vi "Configure Sweep Characteristics.vi"(0 "VISA resource name":refnum<visa-resource-name>, 1 "Sweep Direction (0: Up)":u16(ring) items=["Up", "Down"], 2 "Sweep Type (0: Step)":u16(ring) items=["Step", "List", "Ramp"], 5 "Sweep Mode (0: Off)":u16(ring) items=["Off", "Frequency", "Power", "Frequency and Power"], 7 "Enable Manual Mode (F:Disable)":bool, 9 "Manual Point (1)":i32=1, 11 "error in (no error)":errorcluster, 12 "Manual Frequency (100 kHz)":dbl=100000.0, 13 "Enable Retrace (T:Enable)":bool=TRUE) -> (4 "VISA resource name out":refnum<visa-resource-name>, 15 "error out":errorcluster)   [LabVIEW 2018, in "Agilent PSG MXG Series.lvlib"]
doc: "Configures the sweep type, sweep direction, sweep mode and retrace state of the sweep functions."
uses:
  Agilent PSG MXG Series.lvlib
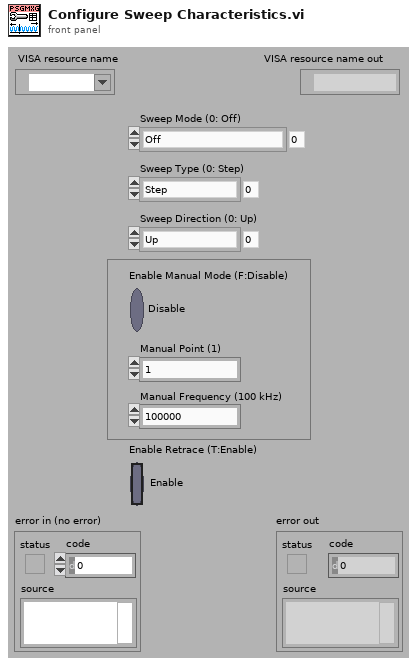
[diagram p1: front panel]
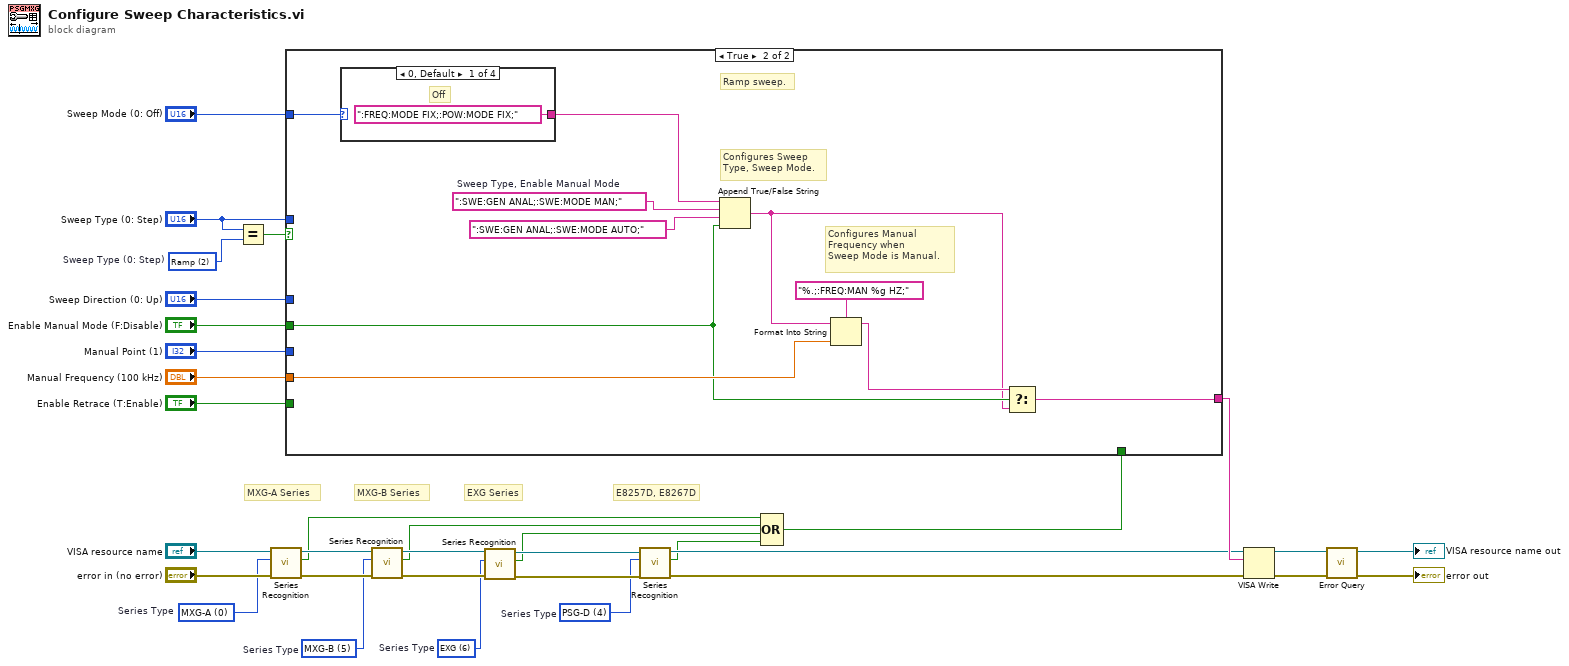
[diagram p0: block diagram]
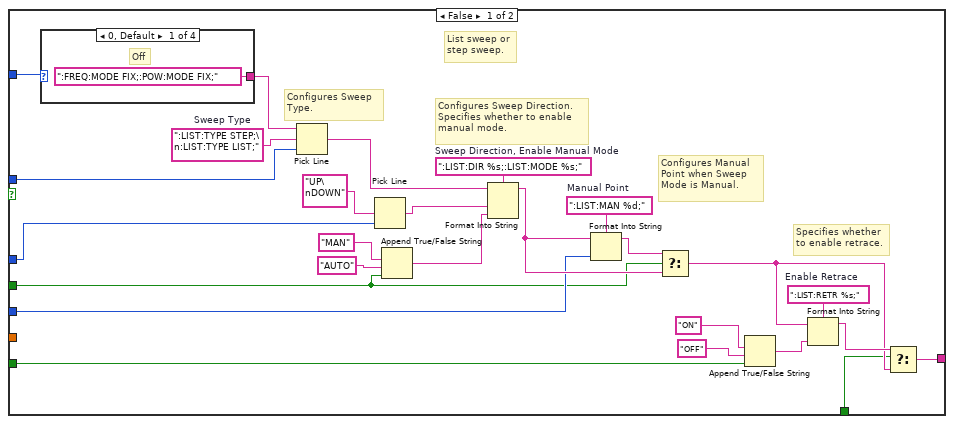
[diagram p2: hidden frame]
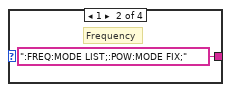
[diagram p3: hidden frame]
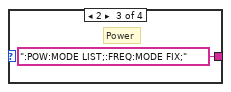
[diagram p4: hidden frame]
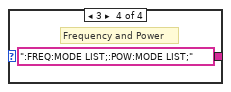
[diagram p5: hidden frame]
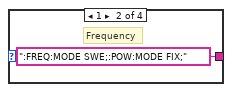
[diagram p6: hidden frame]
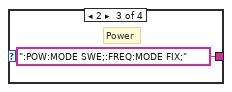
[diagram p7: hidden frame]
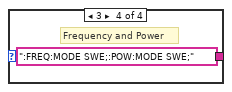
[diagram p8: hidden frame]
diagram:
  w6 = u16 6 items=["MXG-A", "PSG", "PSG-A", "PSG-C", "PSG-D", "MXG-B", "EXG"]  # Series Type
  w7 = u16 5 items=["MXG-A", "PSG", "PSG-A", "PSG-C", "PSG-D", "MXG-B", "EXG"]  # Series Type
  w8 = u16 4 items=["MXG-A", "PSG", "PSG-A", "PSG-C", "PSG-D", "MXG-B", "EXG"]  # Series Type
  w15 = u16 0 items=["MXG-A", "PSG", "PSG-A", "PSG-C", "PSG-D", "MXG-B", "EXG"]  # Series Type
  w33 = 2 items=["Step", "List", "Ramp"]  # Sweep Type (0: Step)
  # "EXG Series"
  # "MXG-B Series"
  # "E8257D, E8267D"
  # "MXG-A Series"
  n1 = Equal?(x="Sweep Type (0: Step)", y=w33) -> (x = y?=w32:bool)
  n2 = call "Series Recognition.vi"("error in (no error)"="error in (no error)", "Series Type (0: MXG)"=w15, "VISA resource name"="VISA resource name") -> ("error out"=w13:errorcluster, "Is Series Correct"=w2:bool, "VISA resource name out"=w14:refnum<visa-resource-name>)  [unwired: 1 in, 5 out]
  n3 = call "Series Recognition.vi"("error in (no error)"=w13, "Series Type (0: MXG)"=w7, "VISA resource name"=w14) -> ("error out"=w10:errorcluster, "Is Series Correct"=w3:bool, "VISA resource name out"=w12:refnum<visa-resource-name>)  [unwired: 1 in, 5 out]
  n4 = call "Series Recognition.vi"("error in (no error)"=w10, "Series Type (0: MXG)"=w6, "VISA resource name"=w12) -> ("error out"=w9:errorcluster, "Is Series Correct"=w4:bool, "VISA resource name out"=w11:refnum<visa-resource-name>)  [unwired: 1 in, 5 out]
  n5 = call "Series Recognition.vi"("error in (no error)"=w9, "Series Type (0: MXG)"=w8, "VISA resource name"=w11) -> ("error out"=w21:errorcluster, "Is Series Correct"=w5:bool, "VISA resource name out"=w22:refnum<visa-resource-name>)  [unwired: 1 in, 5 out]
  n6 = Compound Arithmetic op=OR(w2, w3, w4, w5) -> (w1:bool)
  n7 = case shown="True" w32 {
    tunnel: "Sweep Type (0: Step)" -> [w58 _]
    tunnel: "Sweep Direction (0: Up)" -> [w54 _]
    tunnel: "Enable Manual Mode (F:Disable)" -> [w36 w65]
    tunnel: "Manual Point (1)" -> [w42 _]
    tunnel: "Manual Frequency (100 kHz)" -> [_ w72]
    tunnel: [w46 w70] -> w26
    tunnel: "Enable Retrace (T:Enable)" -> [w50 _]
    tunnel: "Sweep Mode (0: Off)" -> [w40 w69]
    tunnel: w1 -> [w34 _]
    frame False {
      w45 = ":LIST:MAN %d;"  # Manual Point
      w52 = ":LIST:RETR %s;"  # Enable Retrace
      w56 = ":LIST:DIR %s;:LIST:MODE %s;"  # Sweep Direction, Enable Manual Mode
      w59 = ":LIST:TYPE STEP;\n:LIST:TYPE LIST;"  # Sweep Type
      # "Specifies whether\nto enable retrace."
      # "Configures Manual\nPoint when Sweep\nMode is Manual."
      # "Configures Sweep Direction.\nSpecifies whether to enable\nmanual mode."
      # "Configures Sweep\nType."
      # "List sweep or\nstep sweep."
      n8 = case shown="0, Default" w40 {
        tunnel: [":FREQ:MODE FIX;:POW:MODE FIX;" ":FREQ:MODE LIST;:POW:MODE FIX;" ":POW:MODE LIST;:FREQ:MODE FIX;" ":FREQ:MODE LIST;:POW:MODE LIST;"] -> w39
        frame 0, Default {
          # "Off"
        }
        frame 1 {
          # "Frequency"
        }
        frame 2 {
          # "Power"
        }
        frame 3 {
          # "Frequency and Power"
        }
      }
      n9 = Pick Line(string ("")=w39, multi-line string=w59, line index=w58) -> (output string=w57:string)
      n10 = Pick Line(multi-line string="UP\nDOWN", line index=w54) -> (output string=w53:string)  [unwired: 1 out]
      n11 = Append True/False String(1:w36, 2:"AUTO" ("false string"), 3:"MAN" ("true string")) -> (0:w35:string)  [unwired: 1 out]
      n12 = Format Into String(format string=w56, initial string=w57, w53, w35) -> (resulting string=w43:string)  [unwired: 1 in, 1 out]
      n13 = Format Into String(format string=w45, initial string=w43, w42) -> (resulting string=w44:string)  [unwired: 1 in, 1 out]
      n14 = Select(t=w44, s=w36, f=w43) -> (s? t:f=w41:string)
      n15 = Append True/False String(1:w50, 2:"OFF" ("false string"), 3:"ON" ("true string")) -> (0:w51:string)  [unwired: 1 out]
      n16 = Format Into String(format string=w52, initial string=w41, w51) -> (resulting string=w47:string)  [unwired: 1 in, 1 out]
      n17 = Select(t=w47, s=w34, f=w41) -> (s? t:f=w46:string)
    }
    frame True {
      w68 = ":SWE:GEN ANAL;:SWE:MODE MAN;"  # Sweep Type, Enable Manual Mode
      # "Configures Manual\nFrequency when\nSweep Mode is Manual."
      # "Configures Sweep\nType, Sweep Mode."
      # "Ramp sweep."
      n18 = case shown="0, Default" w69 {
        tunnel: [":FREQ:MODE FIX;:POW:MODE FIX;" ":FREQ:MODE SWE;:POW:MODE FIX;" ":POW:MODE SWE;:FREQ:MODE FIX;" ":FREQ:MODE SWE;:POW:MODE SWE;"] -> w66
        frame 0, Default {
          # "Off"
        }
        frame 1 {
          # "Frequency"
        }
        frame 2 {
          # "Power"
        }
        frame 3 {
          # "Frequency and Power"
        }
      }
      n19 = Append True/False String(1:w65, 2:":SWE:GEN ANAL;:SWE:MODE AUTO;" ("false string"), 3:w68, 4:w66) -> (0:w64:string)
      n20 = Format Into String(format string="%.;:FREQ:MAN %g HZ;", initial string=w64, w72) -> (resulting string=w71:string)  [unwired: 1 in, 1 out]
      n21 = Select(t=w71, s=w65, f=w64) -> (s? t:f=w70:string)
    }
  }
  n22 = VISA Write(VISA resource name=w22, write buffer=w26, error in (no error)=w21) -> (VISA resource name out=w25:refnum<visa-resource-name>, error out=w24:errorcluster)  [unwired: 1 out]
  n23 = call "Error Query.vi"("error in (no error)"=w24, "VISA resource name"=w25) -> ("error out"=→"error out":errorcluster, "VISA resource name out"=→"VISA resource name out":refnum<visa-resource-name>)  [unwired: 8 out]
